vi "新记录通知-网络版.vi"() -> ()   [LabVIEW 2017]
uses:
  <vilib>/Utility/miscctls.llb/LVRowAndColumnTypeDef.ctl
  <vilib>/Utility/inputDevices.llb/mouseAcquire.vi
panel:
  in  "列表菜单":enum16{"预览", "忽略此条", "删除缓存文件", "复制到剪贴板"}(ring)
  out "点到行列-实时列表":T1 caption="单元格位置"
  in  "device ID":refnum<k1> caption="设备ID"
  in  "新记录":cluster{"新记录列表行":string[], "对应缓存文件":string}[](array[cluster])
  in  "报警记录列表":i32[](listbox)
  in  "忽略全部":bool
  in  "预览全部":bool
  # "双击或右键菜单浏览"
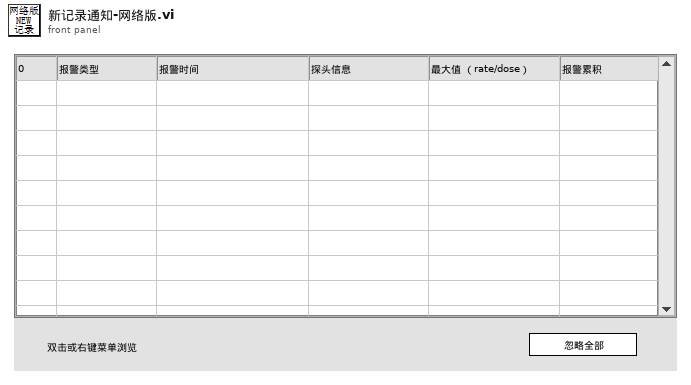
[diagram p1: front panel]
types:
  T1 = typedef "LVRowAndColumnTypeDef.ctl" = cluster{"Row":i32, "Column":i32}
  T2 = enum32{"Invalid", "Standard", "Closed", "Hidden", "Minimized", "Maximized"}
  T3 = typedef "LVPoint32TypeDef.ctl" = cluster{"Horizontal":i32, "Vertical":i32}
  T4 = cluster{"button 1":bool, "button 2":bool, "button 3":bool, "button 4":bool}
  T5 = typedef "eventvkey.ctl" = enum16{"ASCII", "Enter", "Return", "Shift", "Ctrl", "Alt", "Cmd", "Opt", "Caps", "NumLock", "Clear", "Break", "Up", "Down", "Left", "Right", "Insert", "Delete", "Home", "End", "PageUp", "PageDown", "Escape", "Help", "Pause", "ScrollLock", "F1", "F2", "F3", "F4", "F5", "F6", "F7", "F8", "F9", "F10", "F11", "F12", "F13", "F14", "F15", "F16", "F17", "F18", "F19", "F20", "F21", "F22", "F23", "F24", "Play", "VolumeUp", "VolumeDown", "Mute", "Two Byte Char"}
  T6 = cluster{"Shift":bool, "Ctrl":bool, "Alt":bool, "Cmd":bool, "Opt":bool}
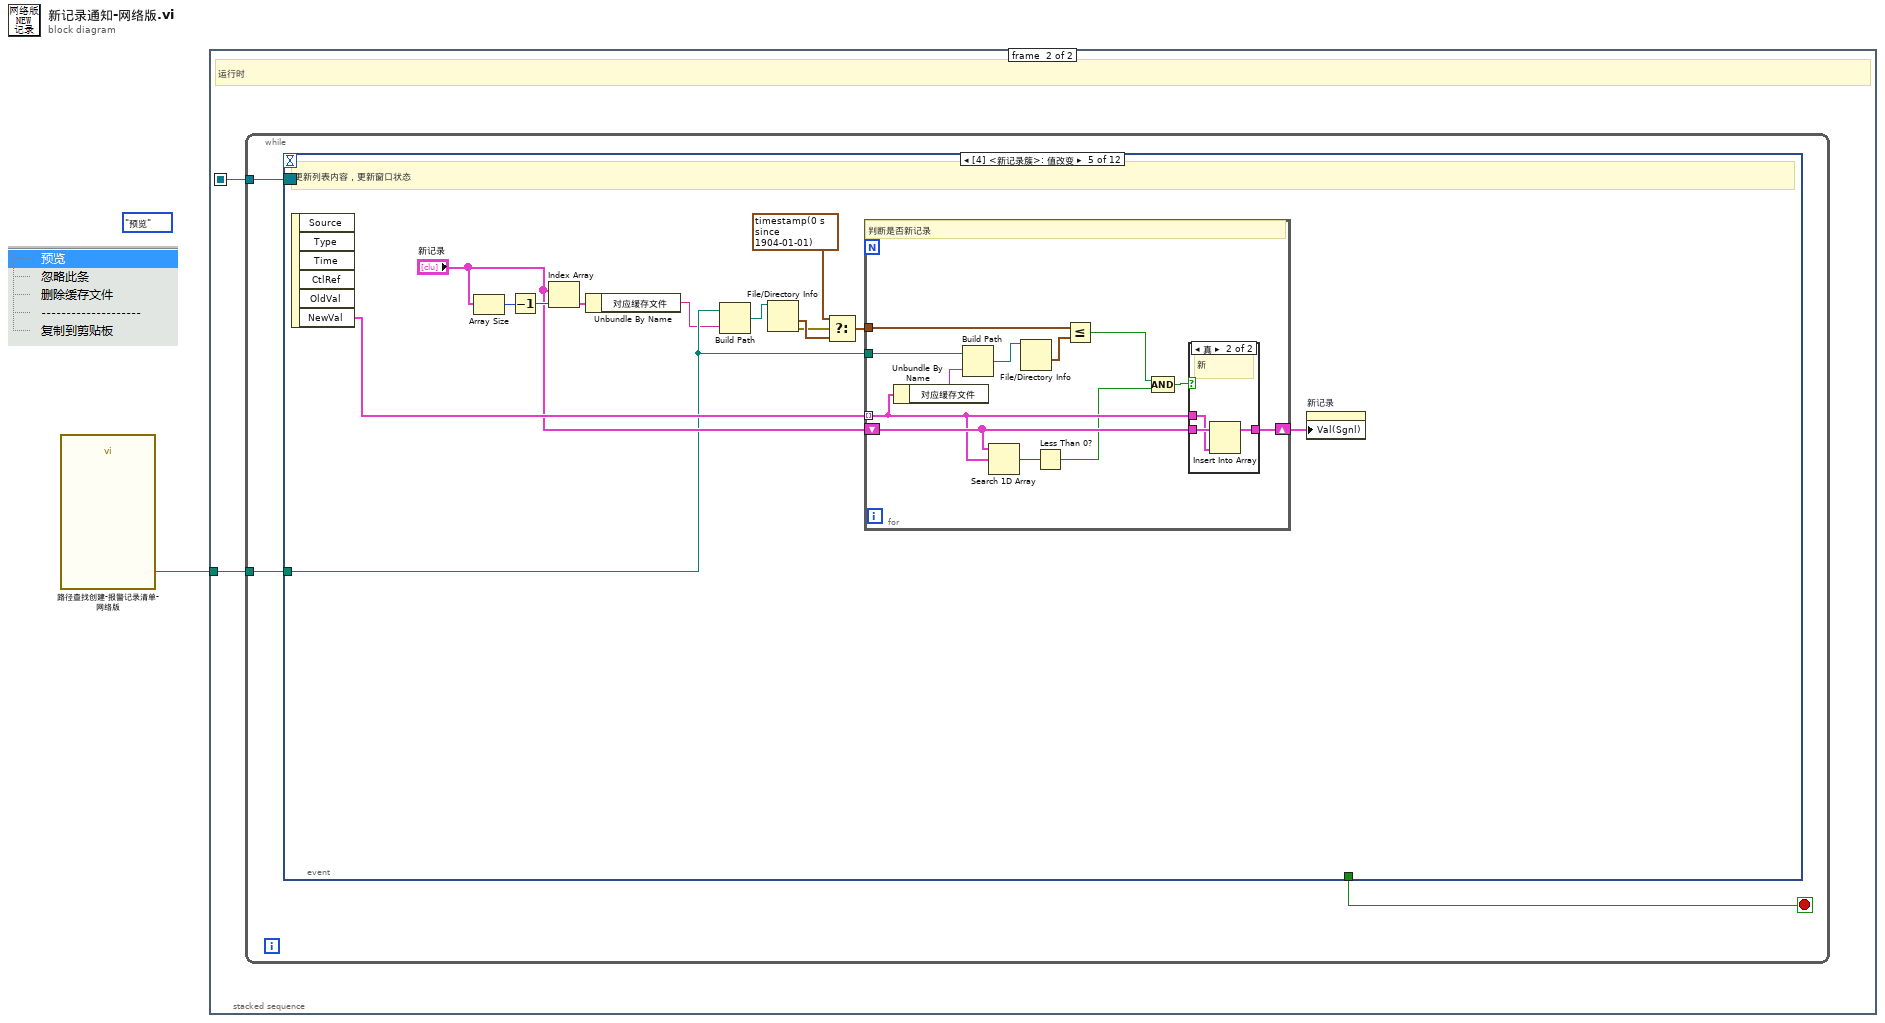
[diagram p0: block diagram]
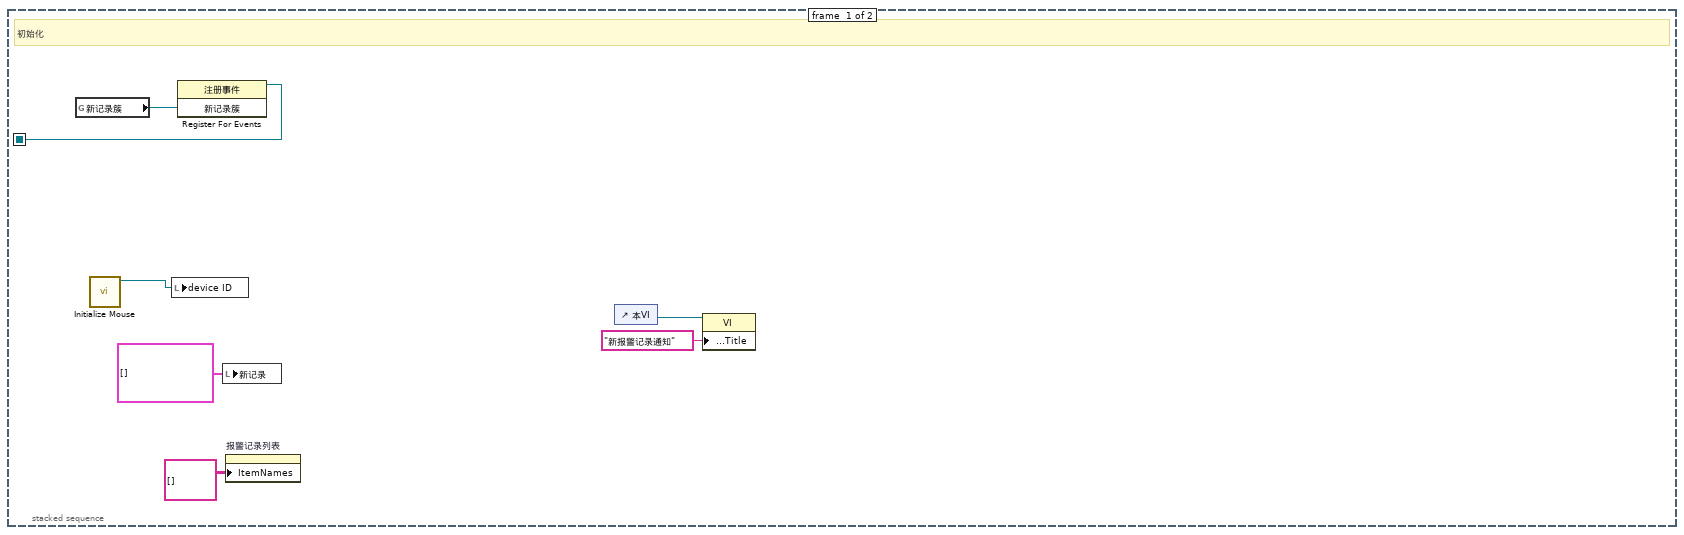
[diagram p2: hidden frame]
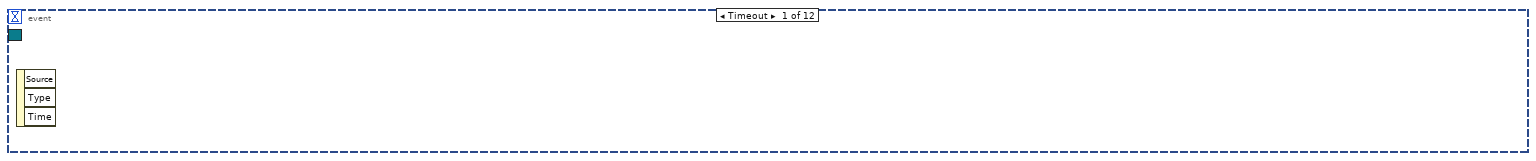
[diagram p3: hidden frame]
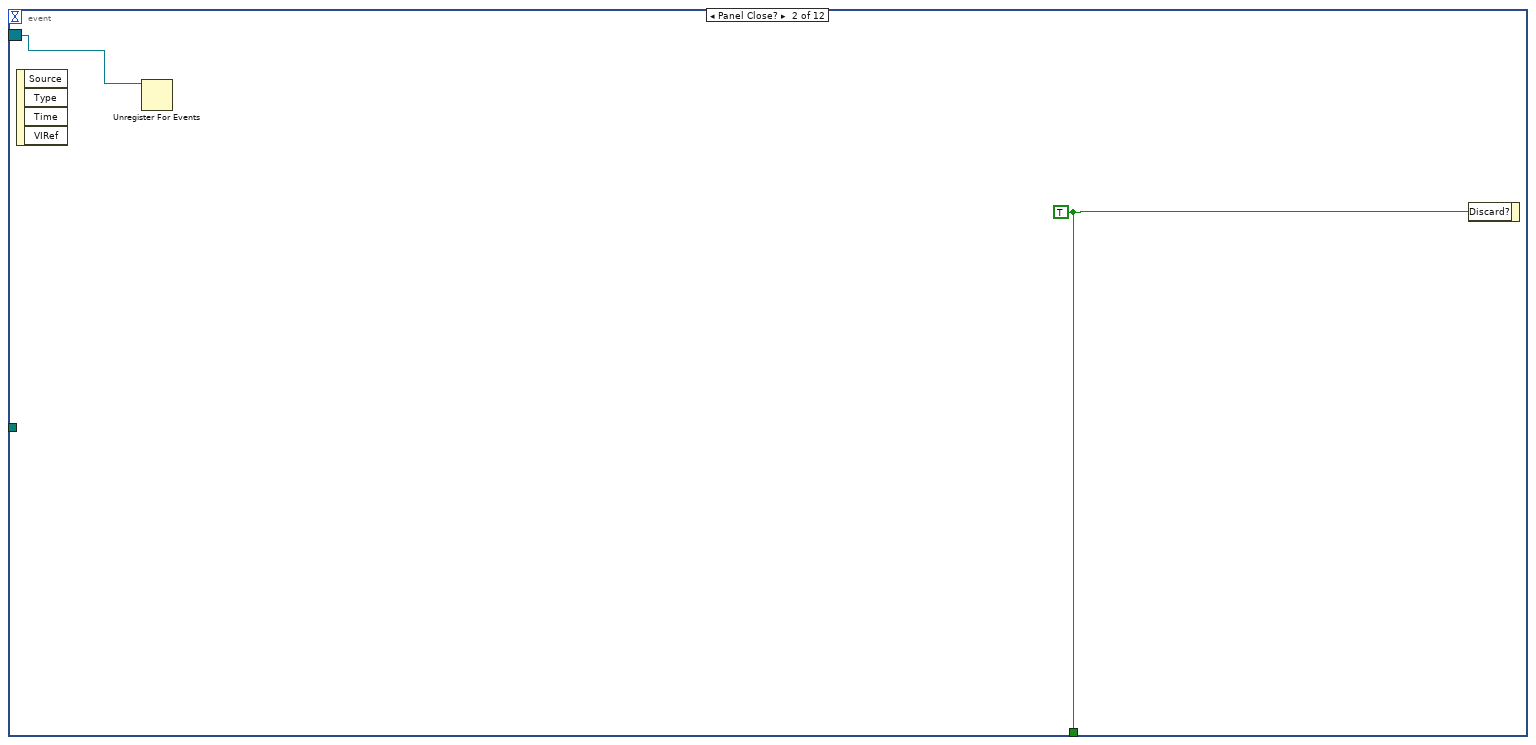
[diagram p4: hidden frame]
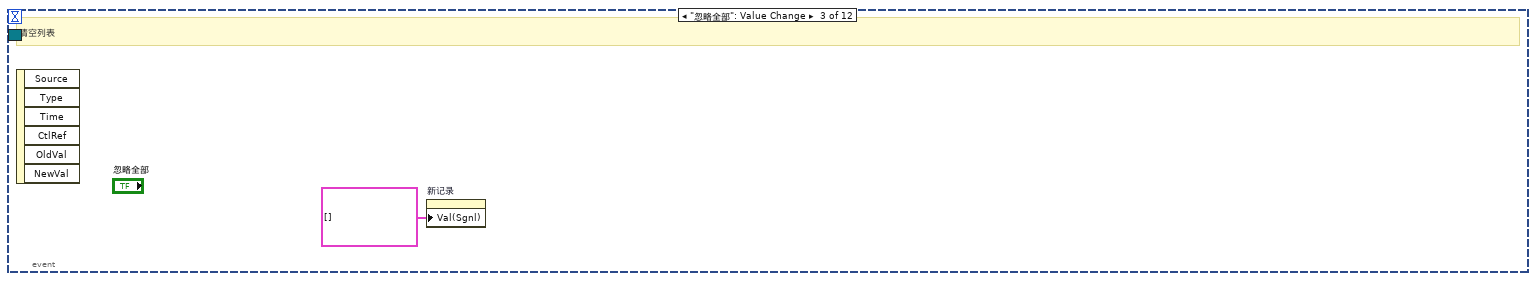
[diagram p5: hidden frame]
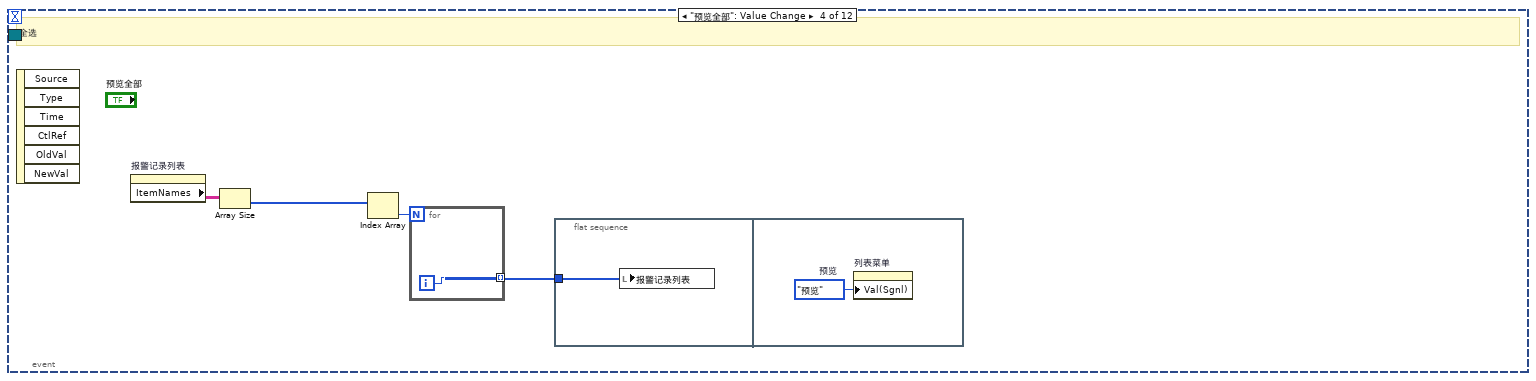
[diagram p6: hidden frame]
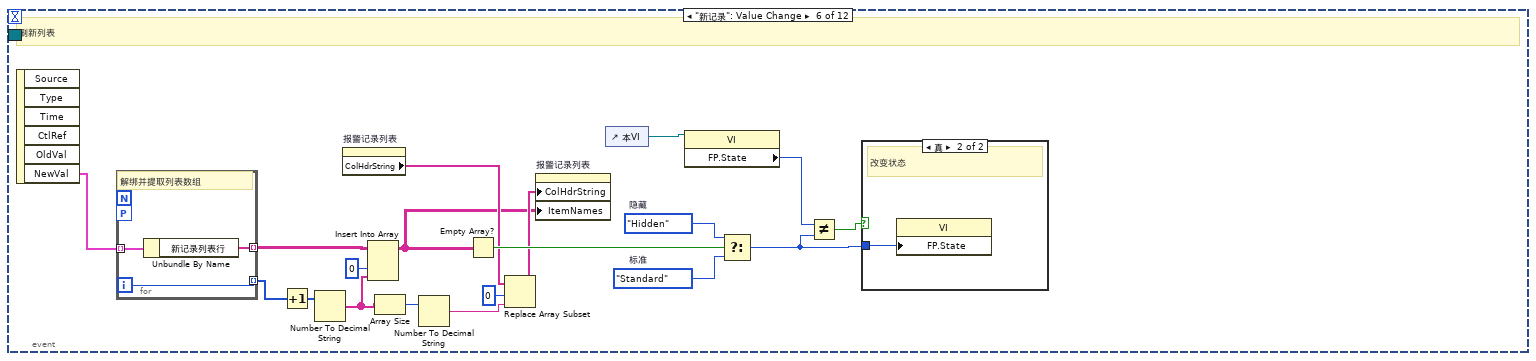
[diagram p8: hidden frame]
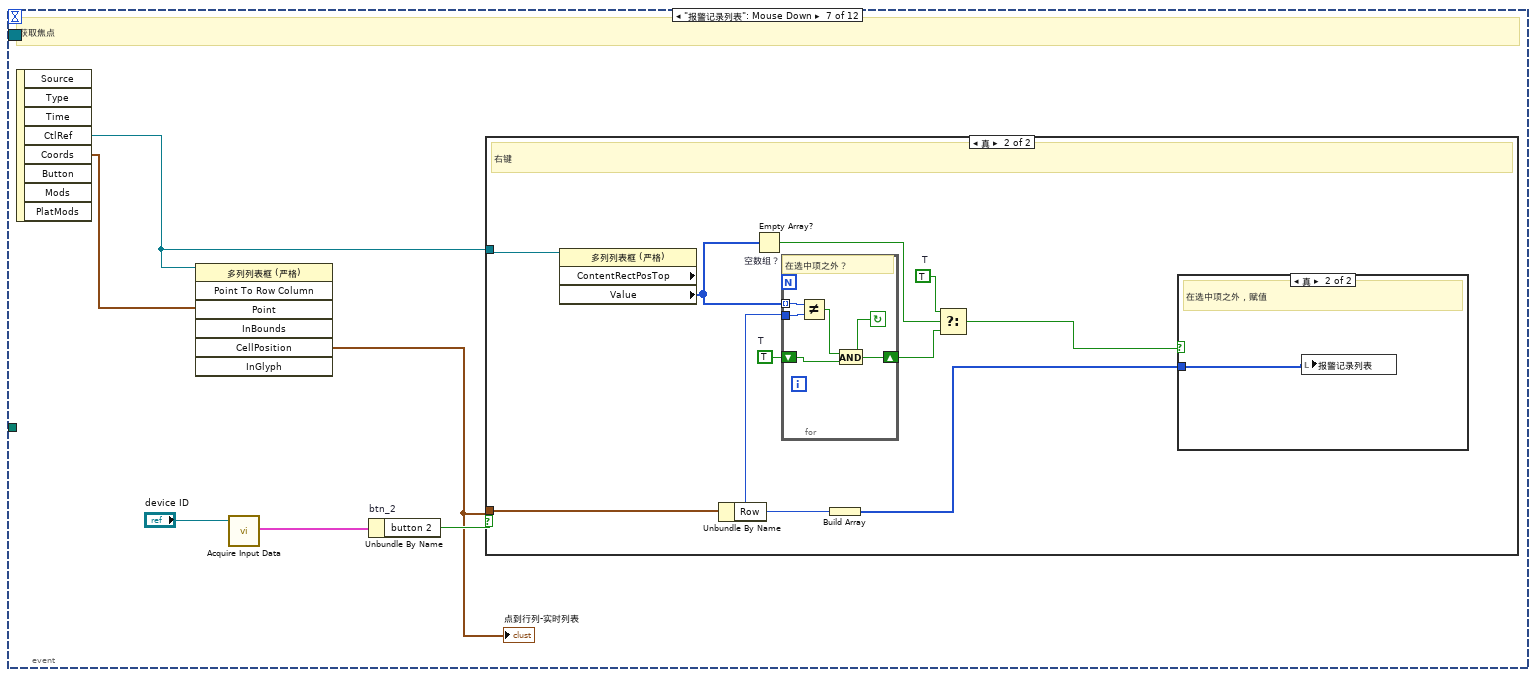
[diagram p10: hidden frame]
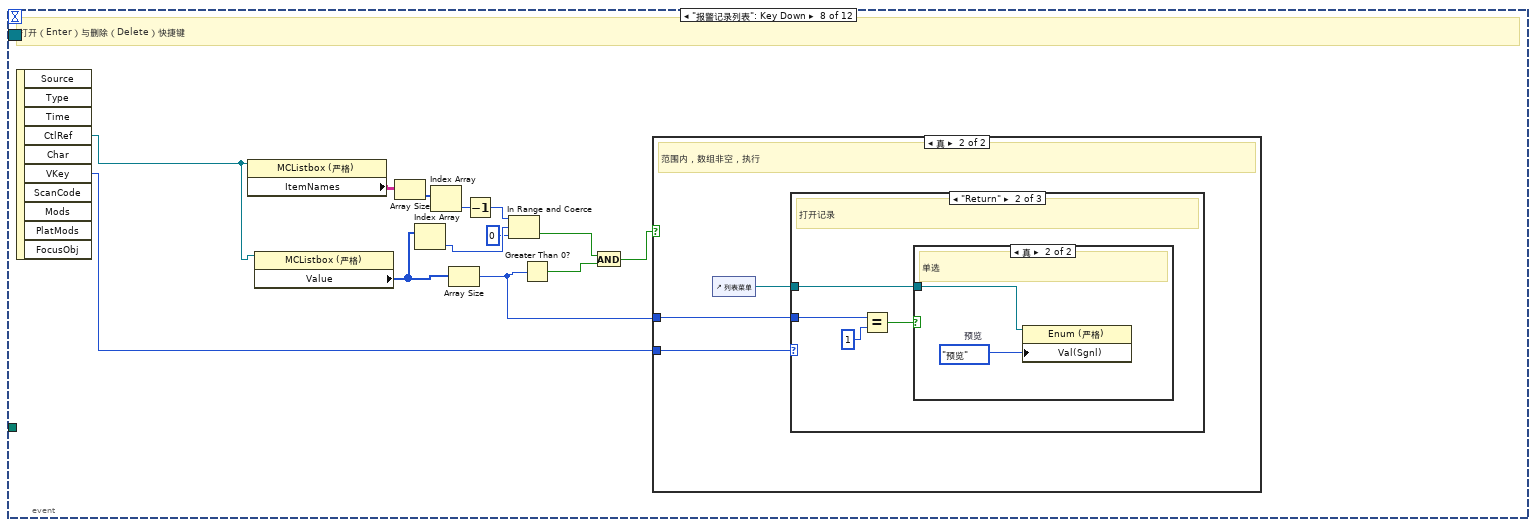
[diagram p13: hidden frame]
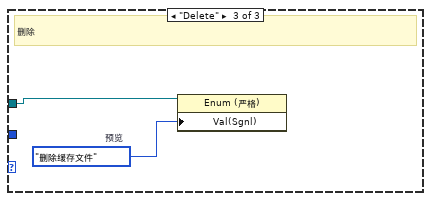
[diagram p17: hidden frame]
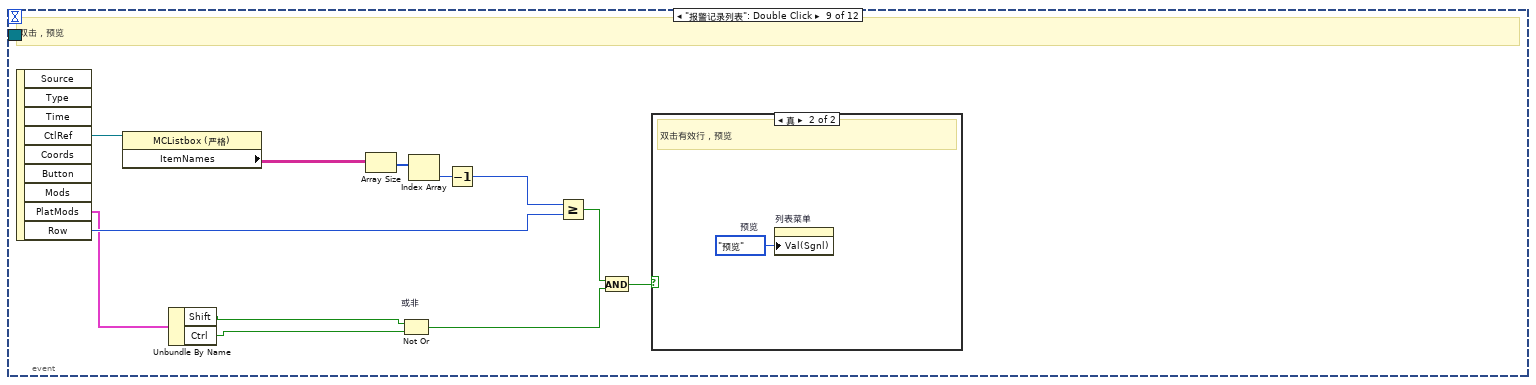
[diagram p18: hidden frame]
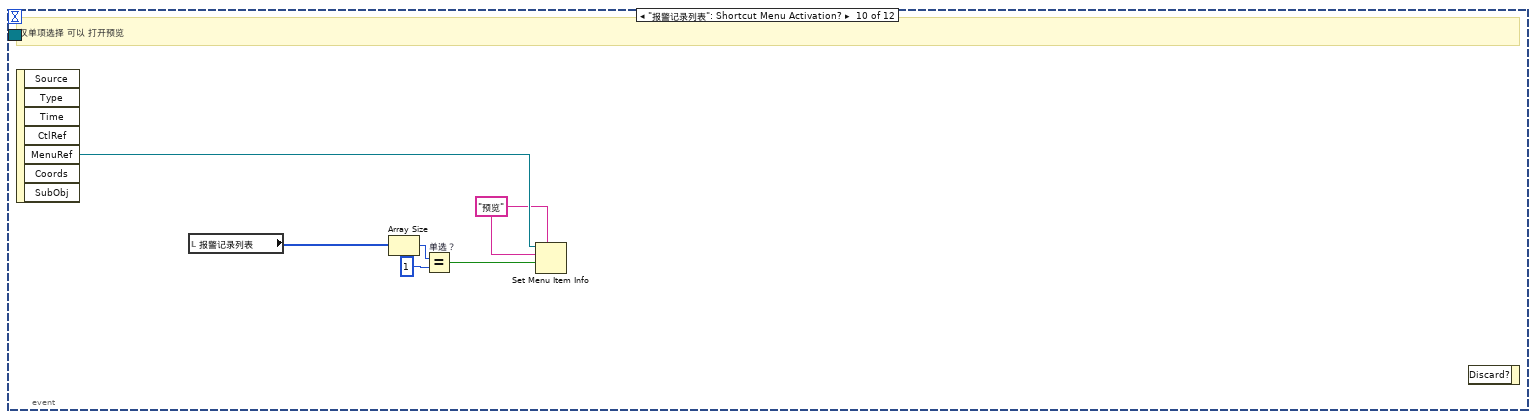
[diagram p20: hidden frame]
diagram:
  (unwired) enum16{"预览", "忽略此条", "删除缓存文件", "复制到剪贴板"}."预览"
  n1 = call "路径查找创建-报警记录清单-网络版.vi"() -> ("缓存数据文件夹"=w1:path)  [unwired: 2 in, 13 out]
  n2 = stacked-sequence {
    seq-local: [w7 _] -> [_ w10]
    tunnel: w1 -> [_ w9]
    frame #0 {
      # "初始化"
      n3 = global read "全局变量-35点监测.vi" "新记录簇"() -> (w8:refnum<vi>)
      n4 = call <vilib>:"Initialize Mouse.vi"() -> ("device ID"=w6:refnum<k1>)  [unwired: 10 in, 1 out]
      n5 = local write "device ID"(w6) -> ()
      n6 = register-events(w8) -> (reference out=w7:refnum<event-registration>)  [unwired: 2 in, 1 out]
      n7 = local write "新记录"(cluster{"新记录列表行":string[], "对应缓存文件":string}[] [] ("新记录")) -> ()
      n8 = property on="报警记录列表" class="MCListbox (严格)"("ItemNames"=string[][] [] ("项名")) -> ()  [unwired: 2 in, 2 out]
      n9 = control-ref of="本VI"() -> (w3:refnum<vi>)
      n10 = property class="VI"(reference=w3, "Front Panel.Title"="新报警记录通知" ("前面板窗口:标题")) -> ()  [unwired: 1 in, 2 out]
    }
    frame #1 {
      # "运行时"
      n11 = while {
        tunnel: w10 -> [w12]
        tunnel: w9 -> [w11]
        stop <- w13 stop-if-true
        n12 = event shown="[4] <新记录簇>: 值改变" {
          selector: w12 -> [_ w14 _ _ _ _ _ _ _ _ _ _]
          dyn-events: _ -> [_ _ _ _ _ _ _ _ _ _ _ _]
          timeout: _ -> [_ _ _ _ _ _ _ _ _ _ _ _]
          tunnel: [_ w15 _ _ _ _ _ _ _ _ _ _] -> w13
          tunnel: w11 -> [_ _ _ _ w26 _ _ _ _ _ _ _]
          event Timeout {
            n13 = event-data() -> ()  [unwired: 1 in, 3 out]
          }
          event Panel Close? {
            w15 = TRUE ("放弃？")
            n14 = event-data() -> ()  [unwired: 1 in, 4 out]
            n15 = Unregister For Events(event registration refnum=w14) -> ()  [unwired: 1 in, 1 out]
            n16 = event-data("Discard?"=w15) -> ()  [unwired: 1 in, 1 out]
          }
          event "忽略全部": Value Change {
            # "清空列表"
            n17 = event-data() -> ()  [unwired: 1 in, 6 out]
            n18 = property on="新记录" class="Arr (严格)"("Val(Sgnl)"=cluster{"新记录列表行":string[], "对应缓存文件":string}[] [] ("值(信号)")) -> ()  [unwired: 2 in, 2 out]
          }
          event "预览全部": Value Change {
            # "全选"
            n19 = event-data() -> ()  [unwired: 1 in, 6 out]
            n20 = property on="报警记录列表" class="MCListbox (严格)"() -> ("ItemNames"=w20:string[][])  [unwired: 2 in, 2 out]
            n21 = Array Size(array=w20) -> (size(s)=w19:i32[])
            n22 = Index Array(array=w19) -> (element=w18:i32)  [unwired: 1 in]
            n23 = for {
              N: w18 -> [_]
              tunnel: [w21] -> w17 mode=indexing
              i -> [w21]
            }
            n24 = flat-sequence {
              tunnel: w17 -> [w22]
              frame #0 {
                n25 = local write "报警记录列表"(w22) -> ()
              }
              frame #1 {
                w23 = enum16{"预览", "忽略此条", "删除缓存文件", "复制到剪贴板"}."预览"  # 预览
                n26 = property on="列表菜单" class="Enum (严格)"("Val(Sgnl)"=w23) -> ()  [unwired: 2 in, 2 out]
              }
            }
          }
          event Value Change {
            # "更新列表内容，更新窗口状态"
            n27 = event-data() -> ("NewVal"=w35:cluster{"新记录列表行":string[], "对应缓存文件":string}[])  [unwired: 1 in, 5 out]
            n28 = Array Size(array="新记录") -> (size(s)=w34:i32)
            n29 = Decrement(x=w34) -> (x-1=w36:i32)
            n30 = Index Array(array="新记录", index=w36) -> (element=w33:cluster{"新记录列表行":string[], "对应缓存文件":string})
            n31 = Unbundle By Name(w33) -> ("对应缓存文件"=w25:string)
            n32 = Build Path(base path=w26, name or relative path=w25) -> (appended path=w27:path)
            n33 = File/Directory Info(path=w27) -> (last mod=w29:timestamp, error out=w24:errorcluster)  [unwired: 1 in, 5 out]
            n34 = Select(t=timestamp(0 s since 1904-01-01) ("上次修改"), s=w24, f=w29) -> (s? t:f=w28:timestamp)
            n35 = for {
              tunnel: w35 -> [w42] mode=indexing
              tunnel: w28 -> [w48]
              shift-right: [w46] -> w31
              shift-left: "新记录" -> [w43]
              tunnel: w26 -> [w38]
              # "判断是否新记录"
              n36 = Unbundle By Name(w42) -> ("对应缓存文件"=w39:string)
              n37 = Build Path(base path=w38, name or relative path=w39) -> (appended path=w37:path)
              n38 = Search 1D Array(1D array=w43, element=w42) -> (index of element=w41:i32)  [unwired: 1 in]
              n39 = File/Directory Info(path=w37) -> (last mod=w44:timestamp)  [unwired: 1 in, 6 out]
              n40 = Less Than 0?(x=w41) -> (x < 0?=w40:bool)
              n41 = Less Or Equal?(x=w48, y=w44) -> (x <= y?=w47:bool)
              n42 = Compound Arithmetic op=AND ("复合运算")(w47, w40) -> (w45:bool)
              n43 = case shown="真" w45 {
                tunnel: w43 -> [w49 w52]
                tunnel: w42 -> [_ w51]
                tunnel: [w49 w50] -> w46
                frame False {
                  # "非新"
                }
                frame True {
                  # "新"
                  n44 = Insert Into Array(array=w52, new element=w51) -> (w50:cluster{"新记录列表行":string[], "对应缓存文件":string}[])  [unwired: 1 in]
                }
              }
            }
            n45 = property on="新记录" class="Arr (严格)"("Val(Sgnl)"=w31) -> ()  [unwired: 2 in, 2 out]
          }
          event "新记录": Value Change {
            w70 = T2."Hidden"  # 隐藏
            w69 = T2."Standard"  # 标准
            # "刷新列表"
            n46 = event-data() -> ("NewVal"=w71:cluster{"新记录列表行":string[], "对应缓存文件":string}[])  [unwired: 1 in, 5 out]
            n47 = for {
              workers-P: _ -> [_]
              tunnel: w71 -> [w75] mode=indexing
              tunnel: [w74] -> w53 mode=indexing
              tunnel: [w73] -> w57 mode=indexing
              i -> [w73]
              # "解绑并提取列表数组"
              n48 = Unbundle By Name(w75) -> ("新记录列表行"=w74:string[])
            }
            n49 = Increment(x=w57) -> (x+1=w62:i32[])
            n50 = Number To Decimal String(number=w62) -> (decimal integer string=w61:string[])  [unwired: 1 in]
            n51 = property on="报警记录列表" class="MCListbox (严格)"() -> ("ColHdrString"=w56:string[])  [unwired: 2 in, 2 out]
            n52 = Insert Into Array(array=w53, index (col)=0 ("禁用的索引 (列)"), new element=w61) -> (w54:string[][])  [unwired: 1 in]
            n53 = Array Size(array=w61) -> (size(s)=w60:i32)
            n54 = Number To Decimal String(number=w60) -> (decimal integer string=w59:string)  [unwired: 1 in]
            n55 = Empty Array?(array=w54) -> (empty?=w68:bool)
            n56 = Replace Array Subset(array=w56, new element=w59, index=0 ("索引")) -> (w55:string[])
            n57 = property on="报警记录列表" class="MCListbox (严格)"("ColHdrString"=w55, "ItemNames"=w54) -> ()  [unwired: 2 in, 2 out]
            n58 = control-ref of="本VI"() -> (w67:refnum<vi>)
            n59 = property class="VI"(reference=w67) -> ("FP.State"=w66:T2)  [unwired: 1 in, 2 out]
            n60 = Select(t=w70, s=w68, f=w69) -> (s? t:f=w65:T2)
            n61 = Not Equal?(x=w66, y=w65) -> (x != y?=w64:bool)
            n62 = case shown="真" w64 {
              tunnel: w65 -> [_ w72]
              frame False {
                # "状态不变"
              }
              frame True {
                # "改变状态"
                n63 = property class="VI"("FP.State"=w72) -> ()  [unwired: 2 in, 2 out]
              }
            }
          }
          event "报警记录列表": Mouse Down {
            # "获取焦点"
            n64 = event-data() -> ("CtlRef"=w77:refnum<vi>, "Coords"=w78:T3)  [unwired: 1 in, 6 out]
            n65 = invoke class="多列列表框 (严格)" method="Point To Row Column"(reference=w77, "Point"=w78) -> ("CellPosition"=w76:T1)  [unwired: 5 in, 6 out]
            "点到行列-实时列表" <- w76
            n66 = call-poly <vilib>:"Acquire Input Data.vi"("device ID"="device ID") -> ("button info"=w80:T4)  [unwired: 15 in, 3 out]
            n67 = Unbundle By Name "btn_2"(w80) -> ("button 2"=w81:bool)
            n68 = case shown="真" w81 {
              tunnel: w77 -> [_ w90]
              tunnel: w76 -> [_ w87]
              frame False {
                # "不是右键"
              }
              frame True {
                w84 = TRUE  # T
                w91 = TRUE  # T
                # "右键"
                n69 = property class="多列列表框 (严格)" props=["ContentRectPosTop", "Value"](reference=w90) -> ("Value"=w86:i32[])  [unwired: 1 in, 3 out]
                n70 = Unbundle By Name(w87) -> ("Row"=w89:i32)
                n71 = Empty Array? "空数组？"(array=w86) -> (empty?=w85:bool)
                n72 = for {
                  tunnel: w86 -> [w97] mode=indexing
                  shift-right: [w94] -> w83
                  shift-left: w91 -> [w95]
                  tunnel: w89 -> [w93]
                  stop <- w94 continue-if-true
                  # "在选中项之外？"
                  n73 = Not Equal?(x=w97, y=w93) -> (x != y?=w96:bool)
                  n74 = And(x=w96, y=w95) -> (x .and. y?=w94:bool)
                }
                n75 = Build Array(w89) -> (w88:i32[])
                n76 = Select(t=w84, s=w85, f=w83) -> (s? t:f=w82:bool)
                n77 = case shown="真" w82 {
                  tunnel: w88 -> [_ w92]
                  frame False {
                    # "在选中项之中，不赋值"
                  }
                  frame True {
                    # "在选中项之外，赋值"
                    n78 = local write "报警记录列表"(w92) -> ()
                  }
                }
              }
            }
          }
          event "报警记录列表": Key Down {
            # "打开（Enter）与删除（Delete）快捷键"
            n79 = event-data() -> ("CtlRef"=w101:refnum<vi>, "VKey"=w98:T5)  [unwired: 1 in, 8 out]
            n80 = property class="MCListbox (严格)"(reference=w101) -> ("ItemNames"=w106:string[][])  [unwired: 1 in, 2 out]
            n81 = property class="MCListbox (严格)"(reference=w101) -> ("Value"=w108:i32[])  [unwired: 1 in, 2 out]
            n82 = Array Size(array=w106) -> (size(s)=w105:i32[])
            n83 = Index Array(array=w108) -> (element=w109:i32)  [unwired: 1 in]
            n84 = Index Array(array=w105) -> (element=w104:i32)  [unwired: 1 in]
            n85 = Array Size(array=w108) -> (size(s)=w99:i32)
            n86 = Decrement(x=w104) -> (x-1=w103:i32)
            n87 = In Range and Coerce(upper limit=w103, x=w109, lower limit=0 ("下限")) -> (In Range?=w110:bool)  [unwired: 1 out]
            n88 = Greater Than 0?(x=w99) -> (x > 0?=w102:bool)
            n89 = And(x=w110, y=w102) -> (x .and. y?=w100:bool)
            n90 = case shown="真" w100 {
              tunnel: w99 -> [_ w113]
              tunnel: w98 -> [_ w112]
              frame False {
                # "数组空，不执行"
              }
              frame True {
                # "范围内，数组非空，执行"
                n91 = control-ref of="列表菜单"() -> (w111:refnum<vi>)
                n92 = case shown="\"Return\"" w112 {
                  tunnel: w113 -> [_ w117 _]
                  tunnel: w111 -> [_ w114 w120]
                  frame "ASCII", Default {
                    # "不执行"
                  }
                  frame "Return" {
                    # "打开记录"
                    n93 = Equal?(x=w117, y=1) -> (x = y?=w115:bool)
                    n94 = case shown="真" w115 {
                      tunnel: w114 -> [_ w118]
                      frame False {
                        # "多选"
                      }
                      frame True {
                        w119 = enum16{"预览", "忽略此条", "删除缓存文件", "复制到剪贴板"}."预览"  # 预览
                        # "单选"
                        n95 = property on="属性节点" class="Enum (严格)"(reference=w118, "Val(Sgnl)"=w119) -> ()  [unwired: 1 in, 2 out]
                      }
                    }
                  }
                  frame "Delete" {
                    w121 = enum16{"预览", "忽略此条", "删除缓存文件", "复制到剪贴板"}."删除缓存文件"  # 预览
                    # "删除"
                    n96 = property on="属性节点" class="Enum (严格)"(reference=w120, "Val(Sgnl)"=w121) -> ()  [unwired: 1 in, 2 out]
                  }
                }
              }
            }
          }
          event "报警记录列表": Double Click {
            # "双击，预览"
            n97 = event-data() -> ("CtlRef"=w133:refnum<vi>, "PlatMods"=w125:T6, "Row"=w128:i32)  [unwired: 1 in, 6 out]
            n98 = property class="MCListbox (严格)"(reference=w133) -> ("ItemNames"=w132:string[][])  [unwired: 1 in, 2 out]
            n99 = Unbundle By Name(w125) -> ("Shift"=w124:bool, "Ctrl"=w123:bool)
            n100 = Array Size(array=w132) -> (size(s)=w131:i32[])
            n101 = Not Or "或非"(1:w123, 2:w124) -> (0:w126:bool)
            n102 = Index Array(array=w131) -> (element=w130:i32)  [unwired: 1 in]
            n103 = Decrement(x=w130) -> (x-1=w129:i32)
            n104 = Greater Or Equal?(x=w129, y=w128) -> (x >= y?=w127:bool)
            n105 = And(x=w127, y=w126) -> (x .and. y?=w122:bool)
            n106 = case shown="真" w122 {
              frame False {
                # "无效行"
              }
              frame True {
                w134 = enum16{"预览", "忽略此条", "删除缓存文件", "复制到剪贴板"}."预览"  # 预览
                # "双击有效行，预览"
                n107 = property on="列表菜单" class="Enum (严格)"("Val(Sgnl)"=w134) -> ()  [unwired: 2 in, 2 out]
              }
            }
          }
          event "报警记录列表": Shortcut Menu Activation? {
            w136 = "预览" ("项标识符")
            # "仅单项选择 可以 打开预览"
            n108 = event-data() -> ("MenuRef"=w137:refnum<k9>)  [unwired: 1 in, 6 out]
            n109 = local read "报警记录列表"() -> (w140:i32[])
            n110 = Array Size(array=w140) -> (size(s)=w139:i32)
            n111 = Equal? "单选？"(x=w139, y=1) -> (x = y?=w135:bool)
            n112 = Set Menu Item Info(7:w136, 9:w135, 10:w136, 11:w137) -> ()  [unwired: 3 in, 2 out]
            n113 = event-data() -> ()  [unwired: 2 in, 1 out]
          }
          event "报警记录列表": Shortcut Menu Selection (User) {
            # "触发菜单事件"
            n114 = event-data() -> ("ItemTag"=w142:string)  [unwired: 1 in, 7 out]
            n115 = property on="列表菜单" class="Enum (严格)"() -> ("Strings []"=w143:string[])  [unwired: 2 in, 2 out]
            n116 = for {
              tunnel: w143 -> [w147] mode=indexing
              tunnel: w142 -> [w146]
              tunnel: [w144] -> w141
              i -> [w144]
              stop <- w145 stop-if-true
              # "寻找匹配项"
              n117 = Equal?(x=w147, y=w146) -> (x = y?=w145:bool)
            }
            n118 = property on="列表菜单" class="Enum (严格)"("Val(Sgnl)"=w141) -> ()  [unwired: 2 in, 2 out]
          }
          event "列表菜单": Value Change {
            # "菜单事件"
            n119 = event-data() -> ("NewVal"=w150:enum16{"预览", "忽略此条", "删除缓存文件", "复制到剪贴板"})  [unwired: 1 in, 5 out]
            n120 = local read "新记录"() -> (w148:cluster{"新记录列表行":string[], "对应缓存文件":string}[])
            n121 = case shown="\"复制到剪贴板\"" w150 {
              tunnel: "报警记录列表" -> [w154 w217 w222 w258]
              tunnel: w148 -> [w158 w215 w223 _]
              frame "预览", Default {
                # "打开预览窗口"
                n122 = property on="报警记录列表" class="MCListbox (严格)"() -> ("ItemNames"=w155:string[][])  [unwired: 2 in, 2 out]
                n123 = Array Size(array=w155) -> (size(s)=w156:i32[])
                n124 = Index Array(array=w154) -> (element=w153:i32)  [unwired: 1 in]
                n125 = Increment(x=w153) -> (x+1=w152:i32)
                n126 = Index Array(array=w156) -> (element=w157:i32)  [unwired: 1 in]
                n127 = Greater Or Equal? "有效行？"(x=w157, y=w152) -> (x >= y?=w151:bool)
                n128 = case shown="真" w151 {
                  tunnel: w154 -> [_ w160]
                  tunnel: w158 -> [_ w159]
                  frame False {
                  }
                  frame True {
                    n129 = stacked-sequence {
                      tunnel: w160 -> [w162 _]
                      tunnel: w159 -> [w161 _]
                      frame #0 {
                        # "打开预览"
                        n130 = call "路径查找创建-报警记录清单-网络版.vi"() -> ("缓存数据文件夹"=w163:path)  [unwired: 2 in, 13 out]
                        n131 = vi-ref "通用报警记录浏览.vi"() -> (w164:refnum<vi>)
                        n132 = disable-structure shown="启用" {
                          disable-tunnel: w164 -> [w168 w187]
                          disable-tunnel: w163 -> [w167 w189]
                          disable-tunnel: w162 -> [w166 w192]
                          disable-tunnel: w161 -> [w165 w193]
                          frame Disabled {
                            # "对于  预分配重入"
                            n133 = for {
                              tunnel: w166 -> [w169] mode=indexing
                              tunnel: w168 -> [w178]
                              tunnel: w167 -> [w175]
                              tunnel: w165 -> [w177]
                              # "打开所有选中项"
                              n134 = Index Array(array=w177, index=w169) -> (element=w176:cluster{"新记录列表行":string[], "对应缓存文件":string})
                              n135 = Unbundle By Name(w176) -> ("对应缓存文件"=w174:string)
                              n136 = Build Path(base path=w175, name or relative path=w174) -> (appended path=w170:path)
                              n137 = Not A Number/Path/Refnum?(number/path/refnum=w170) -> (NaN/Path/Refnum?=w173:bool)
                              n138 = Empty String/Path?(string/path=w170) -> (empty?=w172:bool)
                              n139 = Not Or(1:w172, 2:w173) -> (0:w171:bool)
                              n140 = case shown="真" w171 {
                                tunnel: w178 -> [_ w180]
                                tunnel: w170 -> [_ w179]
                                frame False {
                                # "空路径，非法路径"
                                }
                                frame True {
                                # "有效路径"
                                n141 = property class="VI"(reference=w180) -> ("Name"=w182:string)  [unwired: 1 in, 2 out]
                                n142 = Open VI Reference(type specifier VI Refnum (for type only)=refnum<vi> refnum ("类型说明符VI引用句柄（仅用于类型）"), vi path=w182, options=128 ("选项")) -> (vi reference=w184:refnum<vi>)  [unwired: 3 in, 1 out]
                                n143 = call-by-ref "开始异步调用"(reference=w184, "缓存数据路径"=w179) -> ()  [unwired: 12 in, 2 out]
                                }
                              }
                            }
                          }
                          frame Enabled {
                            # "对于  共享副本重入"
                            n144 = Index Array(array=w192) -> (element=w191:i32)  [unwired: 1 in]
                            n145 = Index Array(array=w193, index=w191) -> (element=w190:cluster{"新记录列表行":string[], "对应缓存文件":string})
                            n146 = Unbundle By Name(w190) -> ("对应缓存文件"=w188:string)
                            n147 = Build Path(base path=w189, name or relative path=w188) -> (appended path=w186:path)
                            n148 = call <vilib>:"Check if File or Folder Exists.vi"("path"=w186) -> ("file or folder exists?"=w185:bool)  [unwired: 8 in, 2 out]
                            n149 = case shown="真" w185 {
                              tunnel: w187 -> [_ w197]
                              tunnel: w186 -> [_ w196]
                              frame False {
                                n150 = call "显示对话框信息2"() -> ("忽略此条"=w194:bool)  [unwired: 10 in, 1 out]
                                n151 = stacked-sequence {
                                tunnel: w194 -> [_]
                                frame #0 {
                                n152 = property on="列表菜单" class="Enum (严格)"("Val(Sgnl)"=enum16{"预览", "忽略此条", "删除缓存文件", "复制到剪贴板"}."忽略此条" ("值(信号)")) -> ()  [unwired: 2 in, 2 out]
                                }
                                }
                              }
                              frame True {
                                # "有效文件"
                                n153 = invoke class="VI" method="FP.Open"(reference=w197, "Activate"=TRUE ("激活？"), "State"=T2."Hidden" ("状态")) -> (reference out=w200:refnum<vi>, error out=w212:errorcluster)  [unwired: 2 in, 3 out]
                                n154 = call "通过控件名获取控件引用.vi"("控件名数组"=string[] ["缓存数据路径"], "VI引用"=w200) -> ("控件引用输出"=w202:refnum<vi>[], "VI引用o"=w204:refnum<vi>)  [unwired: 7 in, 1 out]
                                n155 = Index Array(array=w202) -> (element=w203:refnum<vi>)  [unwired: 1 in]
                                n156 = property class="Ctl"(reference=w203, error in=w212, "Val(Sgnl)"=w196) -> (error out=w213:errorcluster)  [unwired: 1 out]
                                n157 = invoke class="VI" method="Run VI"(reference=w204, error in=w213, "Wait until done"=FALSE ("结束前等待"), "Auto Dispose Ref"=TRUE ("自动销毁引用")) -> (reference out=w207:refnum<vi>, error out=w208:errorcluster)  [unwired: 1 in, 3 out]
                                n158 = invoke class="VI" method="FP.Open"(reference=w207, error in=w208, "Activate"=TRUE ("激活？"), "State"=T2."Standard" ("状态")) -> (error out=w211:errorcluster)  [unwired: 1 in, 4 out]
                                n159 = call <vilib>:"Clear Errors.vi"("error in (no error)"=w211) -> ()  [unwired: 5 in, 2 out]
                              }
                            }
                          }
                        }
                      }
                      frame #1 {
                        # "忽略预览过的记录"
                      }
                    }
                  }
                }
              }
              frame "忽略此条" {
                # "从“新记录”中删除，不删除缓存文件"
                n160 = Reverse 1D Array(array=w217) -> (reversed array=w216:i32[])
                n161 = for {
                  tunnel: w216 -> [w218] mode=indexing
                  shift-right: [w219] -> w214
                  shift-left: w215 -> [w220]
                  # "删除忽略项"
                  n162 = Delete From Array(array=w220, index=w218) -> (array with subset deleted=w219:cluster{"新记录列表行":string[], "对应缓存文件":string}[])  [unwired: 1 in, 1 out]
                }
                n163 = property on="新记录" class="Arr (严格)"("Val(Sgnl)"=w214) -> ()  [unwired: 2 in, 2 out]
              }
              frame "删除缓存文件" {
                # "删除缓存文件，刷新列表"
                n164 = call "显示对话框信息"() -> ("确定"=w221:bool)  [unwired: 10 in, 1 out]
                n165 = case shown="真" w221 {
                  tunnel: w223 -> [_ w225]
                  tunnel: w222 -> [_ w224]
                  frame False {
                    # "取消删除"
                  }
                  frame True {
                    # "确认删除"
                    n166 = stacked-sequence {
                      tunnel: w225 -> [w230 _]
                      tunnel: w224 -> [w229 _]
                      frame #0 {
                        # "删除文件，刷新列表"
                        n167 = call "路径查找创建-报警记录清单-网络版.vi"() -> ("缓存数据文件夹"=w226:path)  [unwired: 2 in, 13 out]
                        n168 = Reverse 1D Array(array=w229) -> (reversed array=w228:i32[])
                        n169 = for {
                          tunnel: w228 -> [w237] mode=indexing
                          shift-right: [w232] -> w227
                          shift-left: w230 -> [w238]
                          tunnel: w226 -> [w231]
                          # "删除文件与列表项"
                          n170 = Delete From Array(array=w238, index=w237) -> (deleted portion=w236:cluster{"新记录列表行":string[], "对应缓存文件":string}, array with subset deleted=w232:cluster{"新记录列表行":string[], "对应缓存文件":string}[])  [unwired: 1 in]
                          n171 = Unbundle By Name(w236) -> ("对应缓存文件"=w235:string)
                          n172 = Build Path(base path=w231, name or relative path=w235) -> (appended path=w233:path)
                          n173 = Delete(path (use dialog)=w233) -> (error out=w234:errorcluster)  [unwired: 4 in, 2 out]
                          n174 = call <vilib>:"Clear Errors.vi"("error in (no error)"=w234) -> ()  [unwired: 5 in, 2 out]
                        }
                        n175 = property on="新记录" class="Arr (严格)"("Val(Sgnl)"=w227) -> ()  [unwired: 2 in, 2 out]
                      }
                      frame #1 {
                        w246 = enum16{"刷新", "预览并生成报表", "删除记录", "复制选中项至剪贴板"}."刷新"  # 刷新
                        # "通知“管理VI”刷新报警记录列表"
                        n176 = vi-ref "多点监测上位机-网络版.vi"() -> (w250:refnum<vi>)
                        n177 = vi-ref "累积剂量查询模块.vi"() -> (w244:refnum<vi>)
                        n178 = call "通过控件名获取控件引用.vi"("控件名数组"=string[] ["信号-刷新"], "VI引用"=w244) -> ("控件引用输出"=w243:refnum<vi>[], "错误输出"=w240:errorcluster)  [unwired: 7 in, 1 out]
                        n179 = call "通过控件名获取控件引用.vi"("控件名数组"=string[] ["菜单项-报警列表"], "VI引用"=w250) -> ("控件引用输出"=w248:refnum<vi>[])  [unwired: 7 in, 2 out]
                        n180 = Index Array(array=w243) -> (element=w242:refnum<vi>)  [unwired: 1 in]
                        n181 = Index Array(array=w248) -> (element=w247:refnum<vi>)  [unwired: 1 in]
                        n182 = property class="Ctl"(reference=w242, error in=w240, "Val(Sgnl)"=TRUE) -> (error out=w239:errorcluster)  [unwired: 1 out]
                        n183 = property class="Ctl"(reference=w247, "Val(Sgnl)"=w246) -> ()  [unwired: 1 in, 2 out]
                        n184 = call <vilib>:"Clear Errors.vi"("error in (no error)"=w239) -> ()  [unwired: 5 in, 2 out]
                      }
                    }
                  }
                }
              }
              frame "复制到剪贴板" {
                w251 = 0 ("禁用的索引 (列)")
                # "筛选选中项，到剪贴板"
                n185 = property on="报警记录列表" class="MCListbox (严格)"() -> ("ItemNames"=w253:string[][], "ColHdrString"=w255:string[])  [unwired: 2 in, 2 out]
                n186 = Delete From Array(array=w253, index (col)=w251) -> (array with subset deleted=w252:string[][])  [unwired: 2 in, 1 out]
                n187 = Delete From Array(array=w255, index=w251) -> (array with subset deleted=w254:string[])  [unwired: 1 in, 1 out]
                n188 = for {
                  tunnel: w252 -> [w269]
                  tunnel: w258 -> [w267] mode=indexing
                  shift-right: [w265] -> w256
                  shift-left: string[][] [] ("ItemNames") -> [w268]
                  # "筛选选中项"
                  n189 = Index Array(array=w269, index (row)=w267) -> (element=w266:string[])  [unwired: 1 in]
                  n190 = Insert Into Array(array=w268, new element=w266) -> (w265:string[][])  [unwired: 2 in]
                }
                n191 = Array To Spreadsheet String(array=w256, 3:"%s" ("格式字符串")) -> (spreadsheet string=w262:string)  [unwired: 1 in]
                n192 = Array To Spreadsheet String(array=w254, 3:"%s" ("格式字符串")) -> (spreadsheet string=w264:string)  [unwired: 1 in]
                n193 = control-ref of="本应用程序"() -> (w260:refnum<vi>)
                n194 = Concatenate Strings(w264, w262) -> (w263:string)
                n195 = invoke class="App" method="Clipboard.Write"(reference=w260, "Param 0"=w263) -> ()  [unwired: 2 in, 4 out]
              }
            }
          }
        }
      }
    }
  }
